vi "Rotate to Deg.vi"(8 "error in (no error)":errorcluster caption="错误输入（无错误）", 9 "Speed":dbl, 10 "Target":dbl, 11 "VISA resource name in":refnum<visa-resource-name> caption="VISA资源名称输入") -> (0 "error out":errorcluster caption="错误输出", 3 "VISA resource name out":refnum<visa-resource-name> caption="VISA资源名称输出")   [LabVIEW 2015]
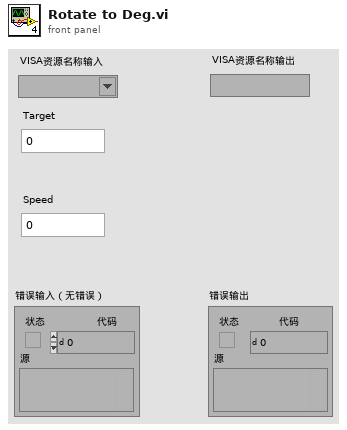
[diagram p1: front panel]
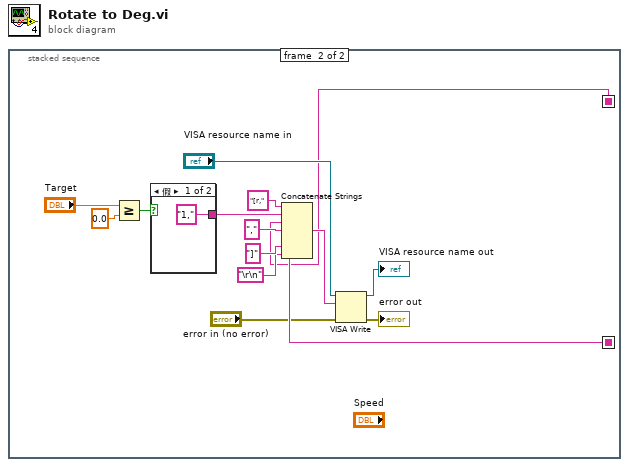
[diagram p0: block diagram]
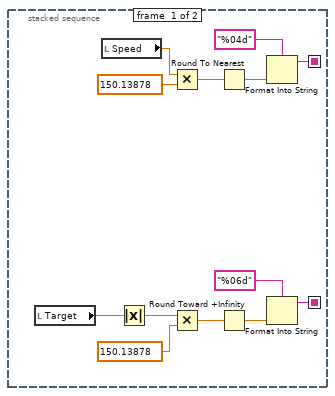
[diagram p2: hidden frame]
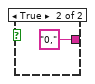
[diagram p3: hidden frame]
diagram:
  n1 = stacked-sequence {
    seq-local: [w3 _] -> [_ w24]
    seq-local: [w1 _] -> [_ w15]
    frame #0 {
      n2 = local read "Target"() -> (w4:dbl)
      n3 = local read "Speed"() -> (w2:dbl)
      n4 = Absolute Value(x=w4) -> (abs(x)=w5:dbl)
      n5 = Multiply(x=w2, y=150.13878) -> (x*y=w12:dbl)
      n6 = Multiply(x=w5, y=150.13878) -> (x*y=w7:dbl)
      n7 = Round To Nearest(number=w12) -> (nearest integer value=w10:dbl)
      n8 = Round Toward +Infinity(x=w7) -> (ceil(x): smallest int >= x=w9:dbl)
      n9 = Format Into String(format string="%04d" ("格式字符串"), w10) -> (resulting string=w1:string)  [unwired: 2 in, 1 out]
      n10 = Format Into String(format string="%06d" ("格式字符串"), w9) -> (resulting string=w3:string)  [unwired: 2 in, 1 out]
    }
    frame #1 {
      n11 = Greater Or Equal?(x="Target", y=0.0) -> (x >= y?=w23:bool)
      n12 = case shown="假" w23 {
        tunnel: ["1," ("字符串") "0," ("字符串")] -> w16
        frame False {
        }
        frame True {
        }
      }
      n13 = Concatenate Strings("[r,", w16, w15, "," ("字符串"), w24, "]" ("字符串"), "\r\n") -> (w20:string)
      n14 = VISA Write(VISA resource name="VISA resource name in", write buffer=w20, error in (no error)="error in (no error)") -> (VISA resource name out=→"VISA resource name out":refnum<visa-resource-name>, error out=→"error out":errorcluster)  [unwired: 1 out]
    }
  }
